vi "DSF Configuration File to Cluster.vi"(8 "error in (no error)":errorcluster, 11 "dsf configuration file path":path) -> (0 "error out":errorcluster, 2 "framework configuration out":T1, 3 "dsf configuration file path dup":path)   [LabVIEW 2017, in "DSF Core.lvlib" / "Configuration Session.lvclass"]
uses:
  Configuration Session.lvclass
  Typedefs/DSF Engine Framework Configuration.ctl
  Typedefs/DSF Engine Plugin Configuration.ctl
  Typedefs/DSF Timing Info.ctl
  Typedefs/DSF Engine Plugin Thread Configuration.ctl
  Typedefs/DSF Settings Info.ctl
  Typedefs/DSF Engine Transfer Group Configuration.ctl
  Typedefs/DSF Direction.ctl
  Typedefs/DSF Engine Transfer Configuration.ctl
  Typedefs/DSF Byte Order.ctl
  Typedefs/DSF Engine Channel Configuration.ctl
  Typedefs/DSF Data Type.ctl
  Typedefs/DSF Timeout Behavior.ctl
  Read All Plugin IDs.vi
  Read Plugin.vi
  Read Settings.vi
  Read Group.vi
  Read Transfer.vi
  Read Channel.vi
  DSF Core.lvlib
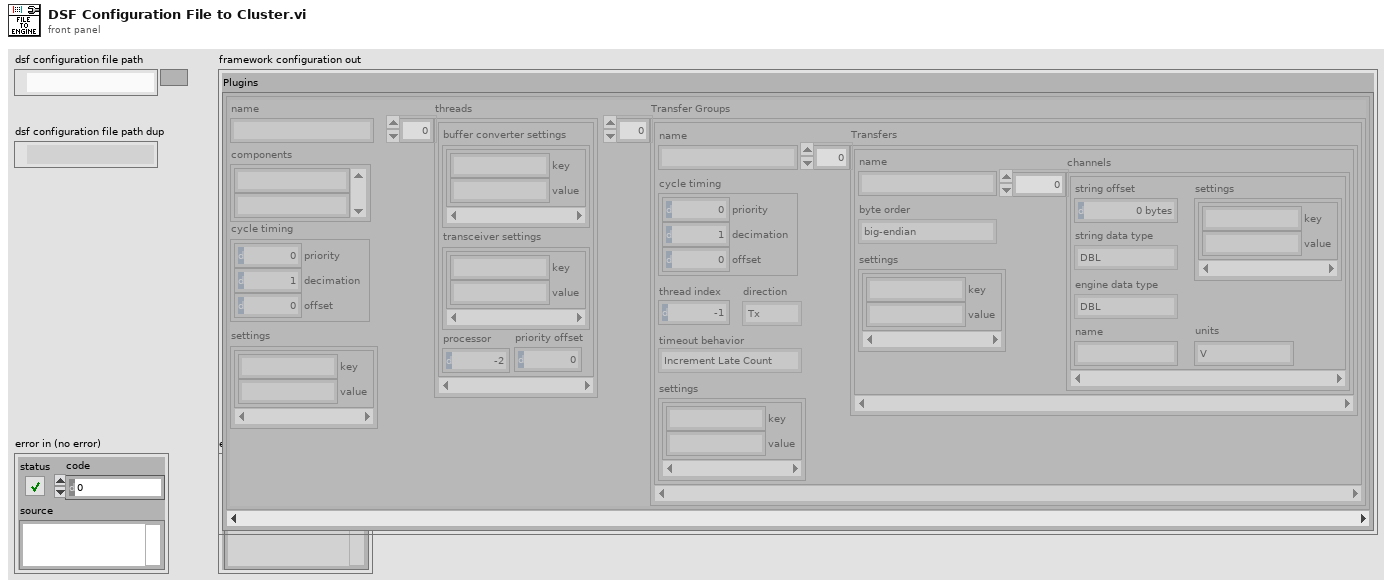
[diagram p1: front panel]
types:
  T1 = typedef "DSF Core.lvlib/DSF Engine Framework Configuration.ctl" = cluster{"Plugins":T2[]}
  T2 = typedef "DSF Core.lvlib/DSF Engine Plugin Configuration.ctl" = cluster{"name":string, "components":string[], "cycle timing":T3, "threads":T4[], "Transfer Groups":T6[], "settings":T5}
  T3 = typedef "DSF Core.lvlib/DSF Timing Info.ctl" = cluster{"priority":u64, "decimation":u64, "offset":u64}
  T4 = typedef "DSF Core.lvlib/DSF Engine Plugin Thread Configuration.ctl" = cluster{"buffer converter settings":T5, "transceiver settings":T5, "processor":i32, "priority offset":i16}
  T5 = typedef "DSF Core.lvlib/DSF Settings Info.ctl" = cluster{"key":string, "value":string}[]
  T6 = typedef "DSF Core.lvlib/DSF Engine Transfer Group Configuration.ctl" = cluster{"name":string, "direction":T7, "cycle timing":T3, "thread index":i32, "settings":T5, "Transfers":T8[], "timeout behavior":T12}
  T7 = typedef "DSF Core.lvlib/DSF Direction.ctl" = enum8{"Tx", "Rx"}
  T8 = typedef "DSF Core.lvlib/DSF Engine Transfer Configuration.ctl" = cluster{"name":string, "byte order":T9, "settings":T5, "channels":T10[]}
  T9 = typedef "DSF Core.lvlib/DSF Byte Order.ctl" = enum8{"big-endian", "little-endian"}
  T10 = typedef "DSF Core.lvlib/DSF Engine Channel Configuration.ctl" = cluster{"string offset":u64, "string data type":T11, "engine data type":T11, "name":string, "settings":T5, "units":string}
  T11 = typedef "DSF Core.lvlib/DSF Data Type.ctl" = enum8{"Bool", "SGL", "DBL", "I8", "I16", "I32", "I64", "U8", "U16", "U32", "U64"}
  T12 = typedef "DSF Core.lvlib/DSF Timeout Behavior.ctl" = enum8{"Increment Late Count", "Throw Error"}
  T13 = typedef "DSF Core.lvlib/DSF Plugin Info.ctl" = cluster{"components":string[], "timing":T3, "group ids":string[], "settings id":string, "threads":T4[]}
  T14 = typedef "DSF Core.lvlib/DSF Group Info.ctl" = cluster{"direction":T7, "timing":T3, "transfer ids":string[], "settings id":string, "thread":i32, "timeout behavior":T12}
  T15 = typedef "DSF Core.lvlib/DSF Transfer Info.ctl" = cluster{"byte order":T9, "channel ids":string[], "settings id":string}
  T16 = typedef "DSF Core.lvlib/DSF Channel Info.ctl" = cluster{"string buffer offset":u64, "string data type":T11, "engine data type":T11, "settings id":string, "units":string}
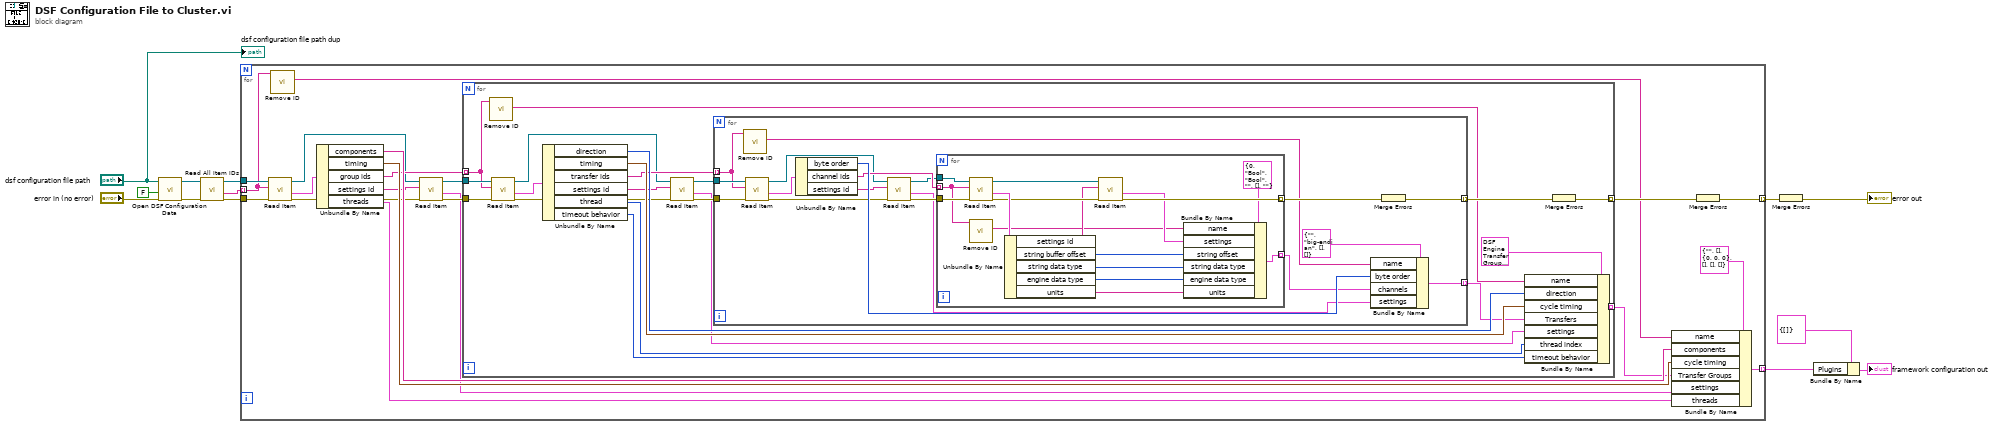
[diagram p0: block diagram]
diagram:
  n1 = call "Open DSF Configuration Data.vi"("error in (no error)"="error in (no error)", "replace if found? (F)"=FALSE ("create file if necessary (T)"), "dsf configuration file path"="dsf configuration file path") -> ("error out"=w4:errorcluster, "Configuration Session"=w5:refnum<class "Configuration Session.lvclass">)  [unwired: 4 in, 3 out]
  n2 = call-poly "Read All Item IDs.vi"("error in (no error)"=w4, "Configuration Session in"=w5) -> ("error out"=w10:errorcluster, "Plugin IDs"=w12:string[], "Configuration Session out"=w11:refnum<class "Configuration Session.lvclass">)  [unwired: 7 in]
  n3 = for {
    tunnel: w12 -> [w15] mode=indexing
    tunnel: w11 -> [w32]
    tunnel: [w28] -> w6 mode=indexing
    tunnel: w10 -> [w21]
    tunnel: [w18] -> w9 mode=indexing
    n4 = call-poly "Read Item.vi"("error in (no error)"=w21, "Plugin ID"=w15, "Configuration Session in"=w32) -> ("error out"=w22:errorcluster, "value"=w31:T13, "Configuration Session out"=w25:refnum<class "Configuration Session.lvclass">)  [unwired: 5 in, 1 out]
    n5 = call "Remove ID.vi"("id string"=w15) -> ("name"=w14:string)  [unwired: 9 in, 1 out]
    n6 = Unbundle By Name(w31) -> ("components"=w30:string[], "timing"=w29:T3, "group ids"=w27:string[], "settings id"=w23:string, "threads"=w17:T4[])
    n7 = call-poly "Read Item.vi"("error in (no error)"=w22, "Settings ID"=w23, "Configuration Session in"=w25) -> ("error out"=w20:errorcluster, "value"=w16:T5, "Configuration Session out"=w24:refnum<class "Configuration Session.lvclass">)  [unwired: 5 in, 1 out]
    n8 = for {
      tunnel: w24 -> [w54]
      tunnel: w27 -> [w34] mode=indexing
      tunnel: [w49] -> w26 mode=indexing
      tunnel: w20 -> [w46]
      tunnel: [w38] -> w19 mode=indexing
      n9 = call "Remove ID.vi"("id string"=w34) -> ("name"=w35:string)  [unwired: 9 in, 1 out]
      n10 = call-poly "Read Item.vi"("error in (no error)"=w46, "Group ID"=w34, "Configuration Session in"=w54) -> ("error out"=w42:errorcluster, "value"=w52:T14, "Configuration Session out"=w45:refnum<class "Configuration Session.lvclass">)  [unwired: 5 in, 1 out]
      n11 = Unbundle By Name(w52) -> ("direction"=w51:T7, "timing"=w50:T3, "transfer ids"=w48:string[], "settings id"=w43:string, "thread"=w37:i32, "timeout behavior"=w36:T12)
      n12 = call-poly "Read Item.vi"("error in (no error)"=w42, "Settings ID"=w43, "Configuration Session in"=w45) -> ("error out"=w41:errorcluster, "value"=w40:T5, "Configuration Session out"=w44:refnum<class "Configuration Session.lvclass">)  [unwired: 5 in, 1 out]
      n13 = for {
        tunnel: w48 -> [w56] mode=indexing
        tunnel: w44 -> [w72]
        tunnel: [w69] -> w47 mode=indexing
        tunnel: w41 -> [w65]
        tunnel: [w58] -> w39 mode=indexing
        n14 = call "Remove ID.vi"("id string"=w56) -> ("name"=w55:string)  [unwired: 9 in, 1 out]
        n15 = call-poly "Read Item.vi"("error in (no error)"=w65, "Transfer ID"=w56, "Configuration Session in"=w72) -> ("error out"=w63:errorcluster, "value"=w71:T15, "Configuration Session out"=w66:refnum<class "Configuration Session.lvclass">)  [unwired: 5 in, 1 out]
        n16 = Unbundle By Name(w71) -> ("byte order"=w70:T9, "channel ids"=w67:string[], "settings id"=w62:string)
        n17 = call-poly "Read Item.vi"("error in (no error)"=w63, "Settings ID"=w62, "Configuration Session in"=w66) -> ("error out"=w61:errorcluster, "value"=w60:T5, "Configuration Session out"=w64:refnum<class "Configuration Session.lvclass">)  [unwired: 5 in, 1 out]
        n18 = for {
          tunnel: [w88] -> w68 mode=indexing
          tunnel: w67 -> [w75] mode=indexing
          tunnel: w64 -> [w87]
          tunnel: w61 -> [w85]
          tunnel: [w82] -> w59 mode=indexing
          n19 = call-poly "Read Item.vi"("error in (no error)"=w85, "Channel ID"=w75, "Configuration Session in"=w87) -> ("error out"=w83:errorcluster, "value"=w86:T16, "Configuration Session out"=w84:refnum<class "Configuration Session.lvclass">)  [unwired: 5 in, 1 out]
          n20 = call "Remove ID.vi"("id string"=w75) -> ("name"=w73:string)  [unwired: 9 in, 1 out]
          n21 = Unbundle By Name(w86) -> ("settings id"=w80:string, "string buffer offset"=w76:u64, "string data type"=w77:T11, "engine data type"=w78:T11, "units"=w74:string)
          n22 = call-poly "Read Item.vi"("error in (no error)"=w83, "Settings ID"=w80, "Configuration Session in"=w84) -> ("error out"=w82:errorcluster, "value"=w79:T5)  [unwired: 5 in, 2 out]
          n23 = Bundle By Name(cluster=T10 {"string offset"=0, "string data type"=enum."Bool", "engine data type"=enum."Bool", "name"="", "settings"=[], "units"=""} ("channel configurations"), "name"=w73, "settings"=w79, "string offset"=w76, "string data type"=w77, "engine data type"=w78, "units"=w74) -> (w88:T10)
        }
        n24 = Bundle By Name(cluster=T8 {"name"="", "byte order"=enum."big-endian", "settings"=[], "channels"=[]} ("Transfer Configuration"), "name"=w55, "byte order"=w70, "channels"=w68, "settings"=w60) -> (w69:T8)
        n25 = Merge Errors(w59) -> (w58:errorcluster)
      }
      n26 = Bundle By Name(cluster=T6 {"name"="", "direction"=enum."Tx", "cycle timing"={"priority"=0, "decimation"=0, "offset"=0}, "thread index"=0, "settings"=[], "Transfers"=[], "timeout behavior"=enum."Increment Late Count"} ("Transfer Group Configuration"), "name"=w35, "direction"=w51, "cycle timing"=w50, "Transfers"=w47, "settings"=w40, "thread index"=w37, "timeout behavior"=w36) -> (w49:T6)
      n27 = Merge Errors(w39) -> (w38:errorcluster)
    }
    n28 = Bundle By Name(cluster=T2 {"name"="", "components"=[], "cycle timing"={"priority"=0, "decimation"=0, "offset"=0}, "threads"=[], "Transfer Groups"=[], "settings"=[]} ("Plugin Configuration"), "name"=w14, "components"=w30, "cycle timing"=w29, "Transfer Groups"=w26, "settings"=w16, "threads"=w17) -> (w28:T2)
    n29 = Merge Errors(w19) -> (w18:errorcluster)
  }
  n30 = Merge Errors(w9) -> (→"error out":errorcluster)
  n31 = Bundle By Name(cluster=T1 {"Plugins"=[]} ("Framework Config (JSON)"), "Plugins"=w6) -> (→"framework configuration out":T1)
  "dsf configuration file path dup" <- "dsf configuration file path"
